vi "LIN LoadLDF.vi"(11 "filepath":path) -> (0 "ResponseSchedule":refnum<k21>, 1 "RequestSchedule":refnum<k21>, 2 "XNET Frame Slave":refnum<k21>, 3 "XNET Frame Master":refnum<k21>)   [LabVIEW 2018]
uses:
  <resource>/objmgr/xnet.rc
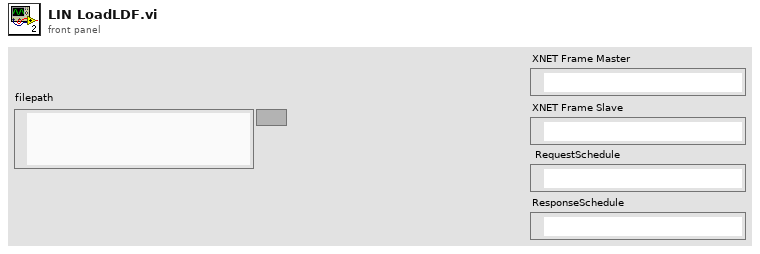
[diagram p1: front panel]
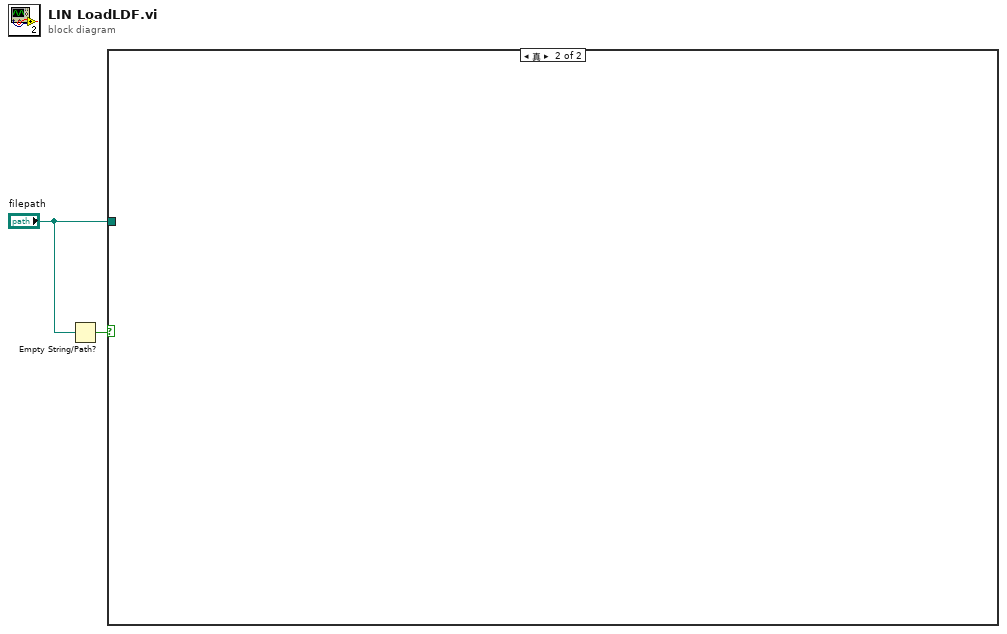
[diagram p0: block diagram]
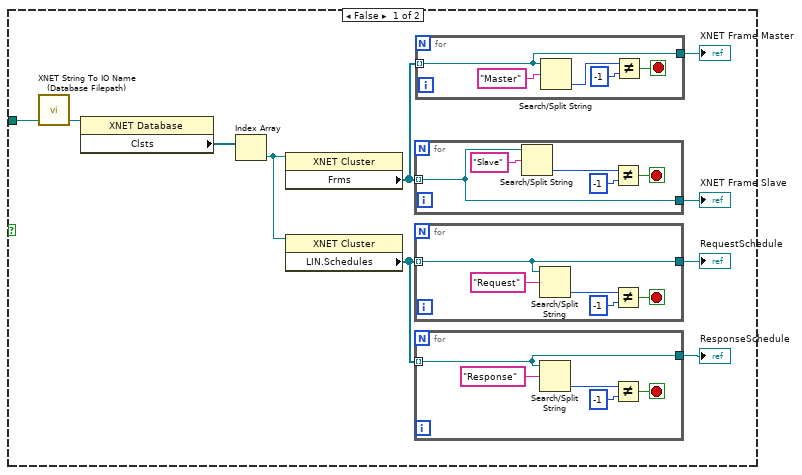
[diagram p2: hidden frame]
diagram:
  n1 = Empty String/Path?(string/path="filepath") -> (empty?=w1:bool)
  n2 = case shown="真" w1 {
    tunnel: "filepath" -> [w10 _]
    frame False {
      n3 = call <vilib>:"XNET String To IO Name (Database Filepath).vi"("filepath"=w10) -> ("XNET Database"=w11:refnum<k21>)  [unwired: 4 in]
      n4 = property class="XNET Database"(reference=w11) -> ("Clsts"=w12:refnum<k21>[])  [unwired: 1 in, 2 out]
      n5 = Index Array(array=w12) -> (element=w3:refnum<k21>)  [unwired: 1 in]
      n6 = property class="XNET Cluster"(reference=w3) -> ("Frms"=w8:refnum<k21>[])  [unwired: 1 in, 2 out]
      n7 = property class="XNET Cluster"(reference=w3) -> ("LIN.Schedules"=w5:refnum<k21>[])  [unwired: 1 in, 2 out]
      n8 = for {
        tunnel: w8 -> [w23] mode=indexing
        tunnel: [w23] -> w7
        stop <- w24 stop-if-true
        n9 = Search/Split String(string=w23, search string/char (-)="Slave" ("搜索字符串/字符(-)")) -> (offset of match=w26:i32)  [unwired: 1 in, 2 out]
        n10 = Not Equal?(x=w26, y=-1) -> (x != y?=w24:bool)
      }
      "XNET Frame Slave" <- w7
      n11 = for {
        tunnel: w5 -> [w18] mode=indexing
        tunnel: [w18] -> w6
        stop <- w19 stop-if-true
        n12 = Search/Split String(string=w18, search string/char (-)="Request" ("搜索字符串/字符(-)")) -> (offset of match=w21:i32)  [unwired: 1 in, 2 out]
        n13 = Not Equal?(x=w21, y=-1) -> (x != y?=w19:bool)
      }
      "RequestSchedule" <- w6
      n14 = for {
        tunnel: w5 -> [w13] mode=indexing
        tunnel: [w13] -> w4
        stop <- w14 stop-if-true
        n15 = Search/Split String(string=w13, search string/char (-)="Response" ("搜索字符串/字符(-)")) -> (offset of match=w16:i32)  [unwired: 1 in, 2 out]
        n16 = Not Equal?(x=w16, y=-1) -> (x != y?=w14:bool)
      }
      "ResponseSchedule" <- w4
      n17 = for {
        tunnel: w8 -> [w28] mode=indexing
        tunnel: [w28] -> w9
        stop <- w29 stop-if-true
        n18 = Search/Split String(string=w28, search string/char (-)="Master" ("搜索字符串/字符(-)")) -> (offset of match=w31:i32)  [unwired: 1 in, 2 out]
        n19 = Not Equal?(x=w31, y=-1) -> (x != y?=w29:bool)
      }
      "XNET Frame Master" <- w9
    }
    frame True {
    }
  }
